vi "demodulate_all.vi"(6 "Config":T5={"I/O"={"Format"={"Rate"=4, "Bits"=32, "Channels"=2}, "card #"=1, "# buffers"=96000}, "High rate STFT"={"Win param"=101.5, "Window type"=61, "Win order"=2, "DFT size"=64, "Channels"=[7], "Oversample"=64}, "Low rate STFT"={"Win param"=120.0, "Window type"=61, "Win order"=8, "DFT size"=64, "Channels"=[7], "Oversample"=64}, "Filtering"={"Hum"={"Frequency"=0.0, "Tc"=0.0, "Limit"=101.5, "FFT filter"=FALSE, "Detrend mode"=enum."Robust linear", "Enable"=FALSE}, "Kalman"={"Process noise"=101.5, "Measure noise"=101.5, "Unlock m noise"=101.5, "Mode"=enum."FFT"}, "Distortion"={"LF cut"=101.5, "Tc"=3.0, "Limit"=101.5, "FFT filter"=FALSE, "Detrend mode"=enum."Robust linear", "Enable"=FALSE}, "Lowpass"={"Frequency"=0.0, "Order"=0, "Enable"=FALSE}, "Impulse"={"Win order"=102, "Locked limit"=101.5, "Locked count"=102, "Threshold Tc"=101.5, "Thresh sigmas"=101.5, "Thresh min"=101.5, "After"=0, "Detrend"=FALSE, "Enable"=FALSE}}} {"Filtering"."Impulse"."Thresh min" format="%#_3p"; "Filtering"."Impulse"."Threshold Tc" format="%#_3p"; "Filtering"."Impulse"."Locked limit" format="%#_3p"; "Filtering"."Impulse"."Thresh sigmas" format="%#_3p"; "Filtering"."Lowpass"."Frequency" format="%#_4p"; "Filtering"."Distortion"."Limit" format="%#_3p"; "Filtering"."Distortion"."LF cut" format="%#_3p"; "Filtering"."Kalman"."Unlock m noise" format="%#_3p"; "Filtering"."Kalman"."Measure noise" format="%#_3p"; "Filtering"."Kalman"."Process noise" format="%#_3p"; "Filtering"."Hum"."Limit" format="%#_3p"; "Filtering"."Hum"."Frequency" format="%#_4p"; "Low rate STFT"."Oversample" min=1 step=1; "Low rate STFT"."Channels" min=0 step=1; "Low rate STFT"."DFT size" min=1 step=1; "Low rate STFT"."Window type" items=["Rectangle"=0, "Hanning"=1, "Hamming"=2, "Blackman-Harris"=3, "Exact Blackman"=4, "Blackman"=5, "Flat Top"=6, "4 Term B-Harris "=7, "7 Term B-Harris"=8, "Low Sidelobe"=9, "Blackman Nuttall"=11, "Triangle"=30, "Bartlett-Hanning"=31, "Bohman"=32, "Parzen"=33, "Welch"=34, "Kaiser"=60, "Dolph-Chebyshev"=61, "Gaussian"=62]; "High rate STFT"."Oversample" min=1 step=1; "High rate STFT"."Channels" min=0 step=1; "High rate STFT"."DFT size" min=1 step=1; "High rate STFT"."Window type" items=["Rectangle"=0, "Hanning"=1, "Hamming"=2, "Blackman-Harris"=3, "Exact Blackman"=4, "Blackman"=5, "Flat Top"=6, "4 Term B-Harris "=7, "7 Term B-Harris"=8, "Low Sidelobe"=9, "Blackman Nuttall"=11, "Triangle"=30, "Bartlett-Hanning"=31, "Bohman"=32, "Parzen"=33, "Welch"=34, "Kaiser"=60, "Dolph-Chebyshev"=61, "Gaussian"=62]}, 7 "Prev carrier amplitudes":cdb[][][](array[numeric]), 9 "Modulation info":T4 {"Hi channels at low" min=0 step=1; "Low carriers" format="%#_6p"; "High carriers" format="%#_6p"}, 10 "Reset":bool, 11 "Raw data":dbl[][](array[numeric])) -> (0 "Unlocked":bool, 1 "Filtered data":dbl[][](array[numeric]), 2 "Trace info out":T1, 3 "High carrier amplitudes":cdb[][][](array[numeric]), 4 "Impulse":bool, 5 "NaN":bool)   [LabVIEW 2014]
uses:
  ilemt_config.ctl
  io_config.ctl
  stft_params.ctl
  <vilib>/Analysis/4window.llb/windowTd.ctl
  filter_params.ctl
  detrend_mode.ctl
  modulation_info.ctl
  trace_info.ctl
  trace_channel.ctl
  ilemt_status.ctl
  <vilib>/Analysis/NI_AALPro.lvlib
panel:
  # "Carrier amplitudes from previous low-rate measurement cycle.  Our interest is with the low carriers, but the whole deal is passed here.  See demod_low.vi for description of carrier amplitudes"
  # "Pages are sensor XYZ axis,\nrows are time (high carrier samples), \ncolumns are high rate source XYZ axis amplitudes."
  # "Our reconstruction of what noiseless input data would have looked like, assuming the carrier ampltude estimates are correct."
  # "Call kf_demodulator on each sensor channel, distributing input data and gathering results."
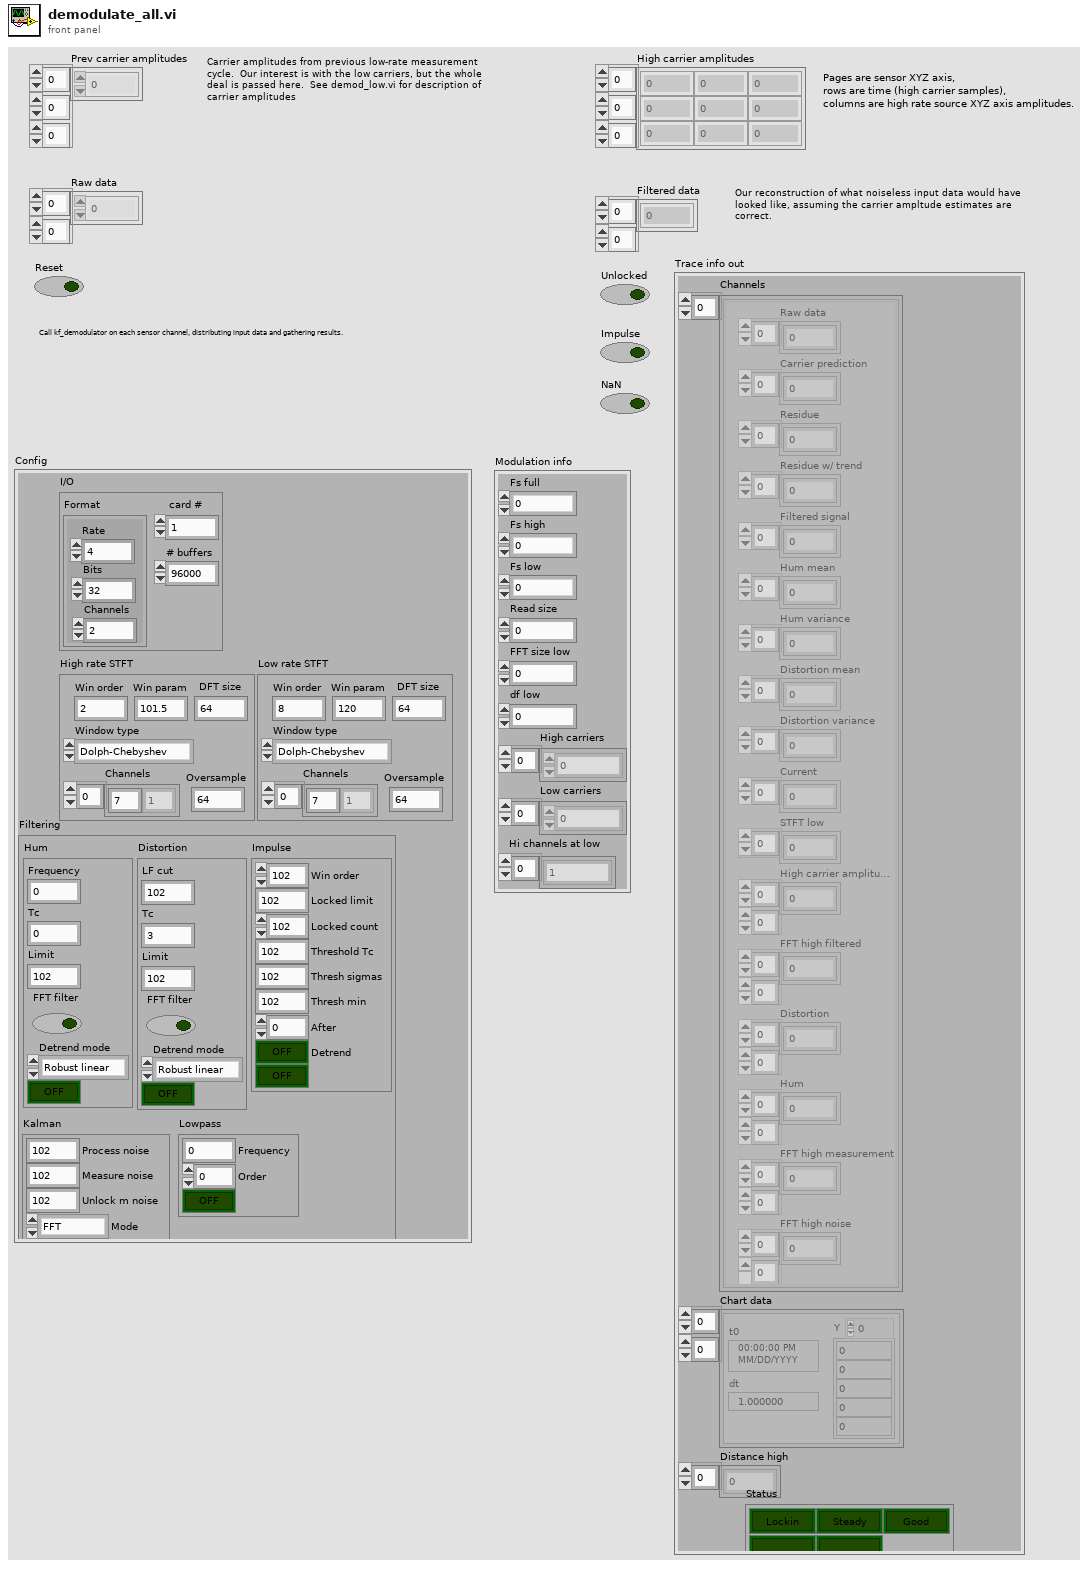
[diagram p1: front panel]
types:
  T1 = typedef "trace_info.ctl" = cluster{"Channels":T2[], "Chart data":waveform(dbl)[][], "Distance high":dbl[], "Status":T3}
  T2 = typedef "trace_channel.ctl" = cluster{"Raw data":dbl[], "Carrier prediction":dbl[], "Residue":dbl[], "Residue w/ trend":dbl[], "Filtered signal":dbl[], "Hum mean":dbl[], "Hum variance":dbl[], "Distortion mean":dbl[], "Distortion variance":dbl[], "Current":dbl[], "STFT low":cdb[], "High carrier amplitudes":cdb[][], "FFT high filtered":cdb[][], "Distortion":cdb[][], "Hum":cdb[][], "FFT high measurement":cdb[][], "FFT high noise":dbl[][]}
  T3 = typedef "ilemt_status.ctl" = cluster{"Unlocked":bool, "Impulse":bool, "NaN":bool, "Backlog":bool, "Clipping":bool}
  T4 = typedef "modulation_info.ctl" = cluster{"Fs full":dbl, "Fs high":dbl, "Fs low":dbl, "Read size":i32, "FFT size low":i32, "df low":dbl, "High carriers":dbl[], "Low carriers":dbl[], "Hi channels at low":i32[]}
  T5 = typedef "ilemt_config.ctl" = cluster{"I/O":T6, "High rate STFT":T7, "Low rate STFT":T7, "Filtering":T9}
  T6 = typedef "io_config.ctl" = cluster{"Format":cluster{"Rate":i32, "Bits":i32, "Channels":u32}, "card #":u32, "# buffers":i32}
  T7 = typedef "stft_params.ctl" = cluster{"Win param":dbl, "Window type":T8, "Win order":i32, "DFT size":i32, "Channels":i32[], "Oversample":i32}
  T8 = typedef "NI_AALPro.lvlib/windowTd.ctl" = u32
  T9 = typedef "filter_params.ctl" = cluster{"Hum":cluster{"Frequency":dbl, "Tc":dbl, "Limit":dbl, "FFT filter":bool, "Detrend mode":T10, "Enable":bool}, "Kalman":cluster{"Process noise":dbl, "Measure noise":dbl, "Unlock m noise":dbl, "Mode":enum16{"FFT", "KF demod"}}, "Distortion":cluster{"LF cut":dbl, "Tc":dbl, "Limit":dbl, "FFT filter":bool, "Detrend mode":T10, "Enable":bool}, "Lowpass":cluster{"Frequency":dbl, "Order":i32, "Enable":bool}, "Impulse":cluster{"Win order":i32, "Locked limit":dbl, "Locked count":i32, "Threshold Tc":dbl, "Thresh sigmas":dbl, "Thresh min":dbl, "After":i32, "Detrend":bool, "Enable":bool}}
  T10 = typedef "detrend_mode.ctl" = enum16{"Zero mean", "Linear", "Robust linear"}
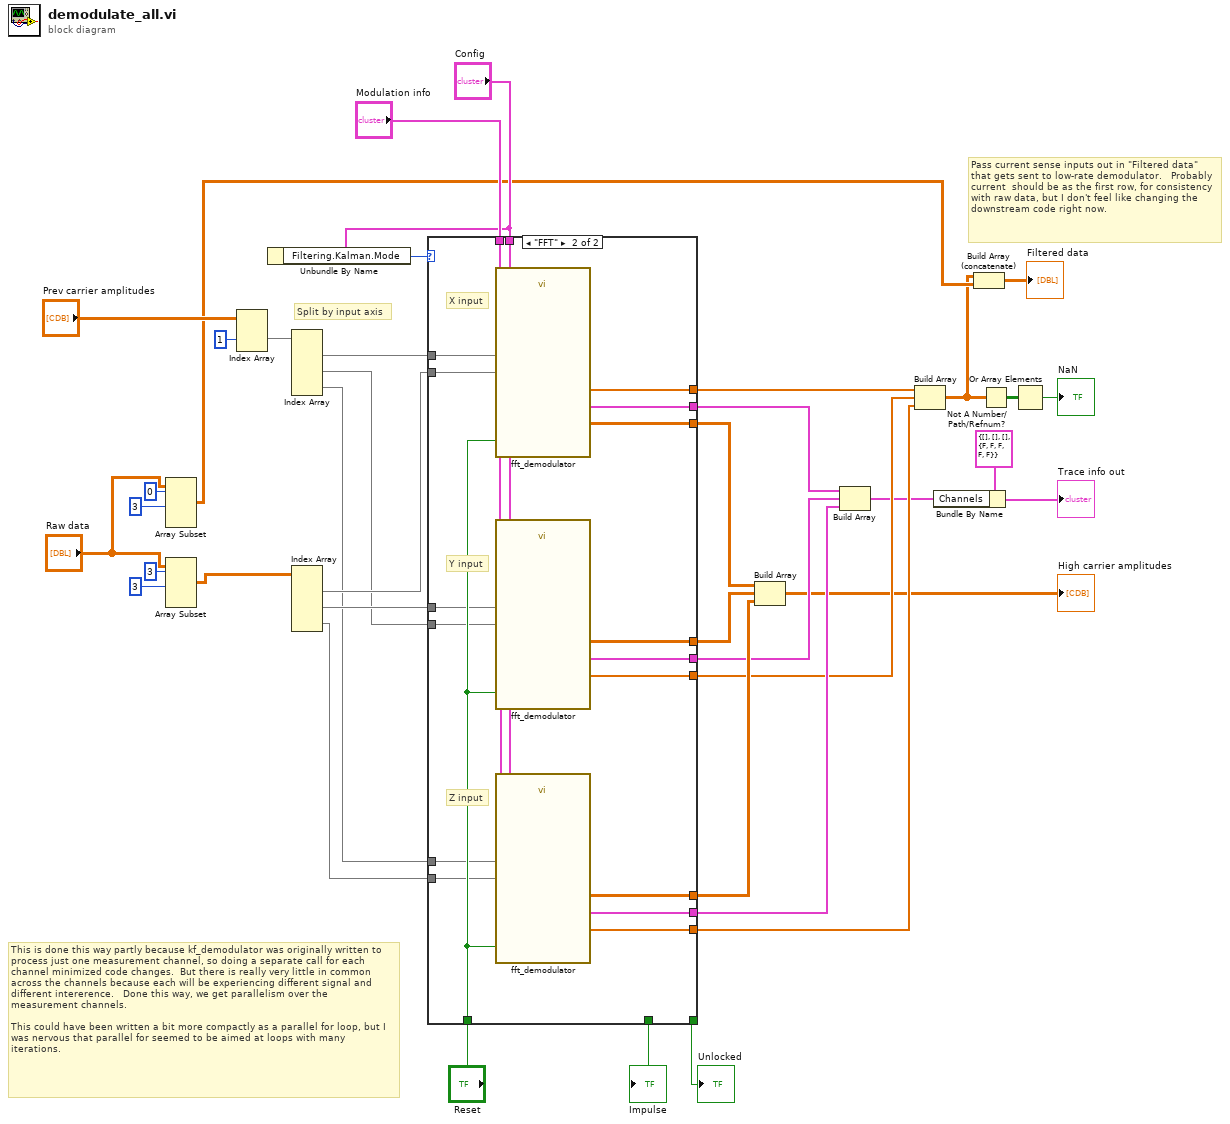
[diagram p0: block diagram]
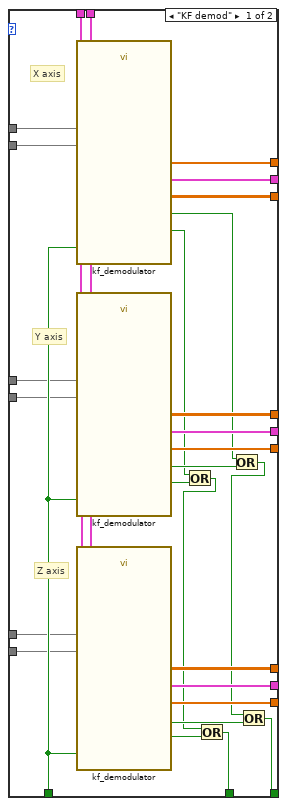
[diagram p2: hidden frame]
diagram:
  # "Split by input axis"
  # "Pass current sense inputs out in \"Filtered data\" that gets sent to low-rate demodulator.   Probably current  should be as the first row, for consistency with raw data, but I don't feel like changing the downstream code right now."
  # "This is done this way partly because kf_demodulator was originally written to process just one measurement channel, so doing a separate call for each channel minimized code changes.  But there is really very little in common across the channels because each will be experiencing different signal and different intererence.   Done this way, we get parallelism over the measurement channels.  \n\nThis could have been written a bit more compactly as a parallel for loop, but I was nervous that parallel for seemed to be aimed at loops with many iterations."
  n1 = Array Subset(array="Raw data", index (row)=0 ("index"), length (row)=3 ("index")) -> (w2:dbl[][])  [unwired: 2 in]
  n2 = Array Subset(array="Raw data", index (row)=3 ("index"), length (row)=3 ("index")) -> (w3:dbl[][])  [unwired: 2 in]
  n3 = Index Array(array="Prev carrier amplitudes", index (dim 1)=1 ("disabled index (row)")) -> (element=w34:cdb[][])  [unwired: 2 in]
  n4 = Unbundle By Name("Config") -> ("Filtering.Kalman.Mode"=w9:enum16{"FFT", "KF demod"})
  n5 = Index Array(array=w34) -> (element #1=w33:cdb[], element #2=w29:cdb[], element #3=w28:cdb[])  [unwired: 6 in]
  n6 = Index Array(array=w3) -> (element #1=w32:dbl[], element #2=w31:dbl[], element #3=w30:dbl[])  [unwired: 6 in]
  n7 = case shown="\"FFT\"" w9 {
    tunnel: "Reset" -> [w67 w85]
    tunnel: "Config" -> [w66 w84]
    tunnel: "Modulation info" -> [w65 w83]
    tunnel: w33 -> [w64 w70]
    tunnel: w32 -> [w63 w82]
    tunnel: w31 -> [w62 w81]
    tunnel: w30 -> [w61 w80]
    tunnel: w29 -> [w60 w69]
    tunnel: w28 -> [w59 w68]
    tunnel: [w58 w79] -> w27
    tunnel: [w57 w78] -> w26
    tunnel: [w56 w77] -> w25
    tunnel: [w55 w76] -> w24
    tunnel: [w54 w75] -> w23
    tunnel: [w53 w74] -> w22
    tunnel: [w52 w73] -> w21
    tunnel: [w51 w72] -> w20
    tunnel: [w50 w71] -> w19
    tunnel: [w41 _] -> w18
    tunnel: [w40 _] -> w17
    frame "KF demod" {
      # "Z axis"
      # "Y axis"
      # "X axis"
      n8 = call "kf_demodulator.vi"("Reset"=w67, "Config"=w66, "Modulation info"=w65, "Low carrier amplitudes"=w64, "Raw data"=w63) -> ("Unlocked"=w48:bool, "Impulse"=w44:bool, "High carrier amplitudes"=w58:cdb[][], "Filtered signal"=w52:dbl[], "Trace info out"=w55:T2)  [unwired: 6 in]
      n9 = call "kf_demodulator.vi"("Reset"=w67, "Config"=w66, "Modulation info"=w65, "Low carrier amplitudes"=w60, "Raw data"=w62) -> ("Unlocked"=w49:bool, "Impulse"=w45:bool, "High carrier amplitudes"=w57:cdb[][], "Filtered signal"=w51:dbl[], "Trace info out"=w54:T2)  [unwired: 6 in]
      n10 = call "kf_demodulator.vi"("Reset"=w67, "Config"=w66, "Modulation info"=w65, "Low carrier amplitudes"=w59, "Raw data"=w61) -> ("Unlocked"=w47:bool, "Impulse"=w43:bool, "High carrier amplitudes"=w56:cdb[][], "Filtered signal"=w50:dbl[], "Trace info out"=w53:T2)  [unwired: 6 in]
      n11 = Or(x=w44, y=w45) -> (x .or. y?=w42:bool)
      n12 = Or(x=w42, y=w43) -> (x .or. y?=w41:bool)
      n13 = Or(x=w48, y=w49) -> (x .or. y?=w46:bool)
      n14 = Or(x=w46, y=w47) -> (x .or. y?=w40:bool)
    }
    frame "FFT" {
      # "Z input"
      # "Y input"
      # "X input"
      n15 = call "fft_demodulator.vi"("Reset"=w85, "Config"=w84, "Modulation info"=w83, "Low carrier amplitudes"=w70, "Raw data"=w82) -> ("High carrier amplitudes"=w79:cdb[][], "Filtered signal"=w73:dbl[], "Trace channel out"=w76:T2)  [unwired: 8 in]
      n16 = call "fft_demodulator.vi"("Reset"=w85, "Config"=w84, "Modulation info"=w83, "Low carrier amplitudes"=w69, "Raw data"=w81) -> ("High carrier amplitudes"=w78:cdb[][], "Filtered signal"=w72:dbl[], "Trace channel out"=w75:T2)  [unwired: 8 in]
      n17 = call "fft_demodulator.vi"("Reset"=w85, "Config"=w84, "Modulation info"=w83, "Low carrier amplitudes"=w68, "Raw data"=w80) -> ("High carrier amplitudes"=w77:cdb[][], "Filtered signal"=w71:dbl[], "Trace channel out"=w74:T2)  [unwired: 8 in]
    }
  }
  "Impulse" <- w18
  "Unlocked" <- w17
  n18 = Build Array(w27, w26, w25) -> (→"High carrier amplitudes":cdb[][][])
  n19 = Build Array(w24, w23, w22) -> (w14:T2[])
  n20 = Build Array(w21, w20, w19) -> (w1:dbl[][])
  n21 = Bundle By Name(cluster=T1 {"Channels"=[], "Chart data"=[], "Distance high"=[], "Status"={"Unlocked"=FALSE, "Impulse"=FALSE, "NaN"=FALSE, "Backlog"=FALSE, "Clipping"=FALSE}} ("Trace info out"), "Channels"=w14) -> (→"Trace info out":T1)
  n22 = Build Array (concatenate)(w1, w2) -> (→"Filtered data":dbl[][])
  n23 = Not A Number/Path/Refnum?(number/path/refnum=w1) -> (NaN/Path/Refnum?=w12:bool[][])
  n24 = Or Array Elements(Boolean array=w12) -> (logical OR=→"NaN":bool)
